vi "ReadQualisysFileInfo.vi"(4 "sortie d'erreur":errorcluster caption="entrée d'erreur", 7 "FichierQualisys":path) -> (0 "error out":errorcluster, 2 "horodatage":timestamp)   [LabVIEW 2015]
uses:
  <vilib>/Utility/miscctls.llb/LVDateTimeRec.ctl
panel:
  out "texte":string
  out "dt":dbl
  out "Freq":u32
  out "Noms des colonnes":string[](array[string])
  out "Noms des bodies":string[](array[string])
  out "NbBodies":u32
  out "NbCameras":u32
  out "NbFrames":u32
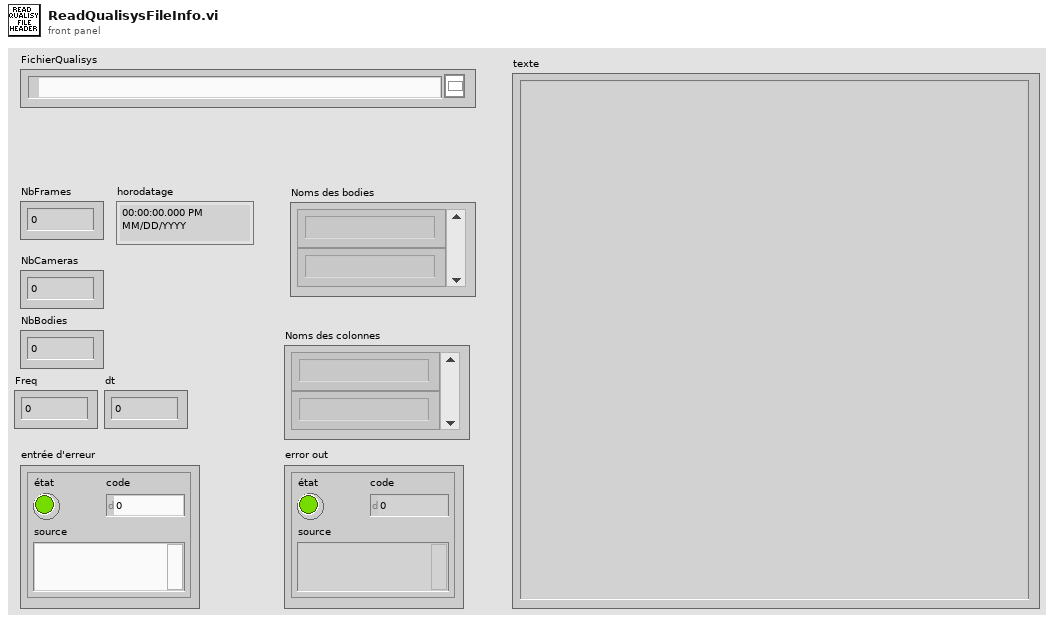
[diagram p1: front panel]
types:
  T1 = typedef "LVDateTimeRec.ctl" = cluster{"fractional second":dbl, "second":i32, "minute":i32, "hour":i32, "day of month":i32, "month":i32, "year":i32, "day of week":i32, "day of year":i32, "DST":i32}
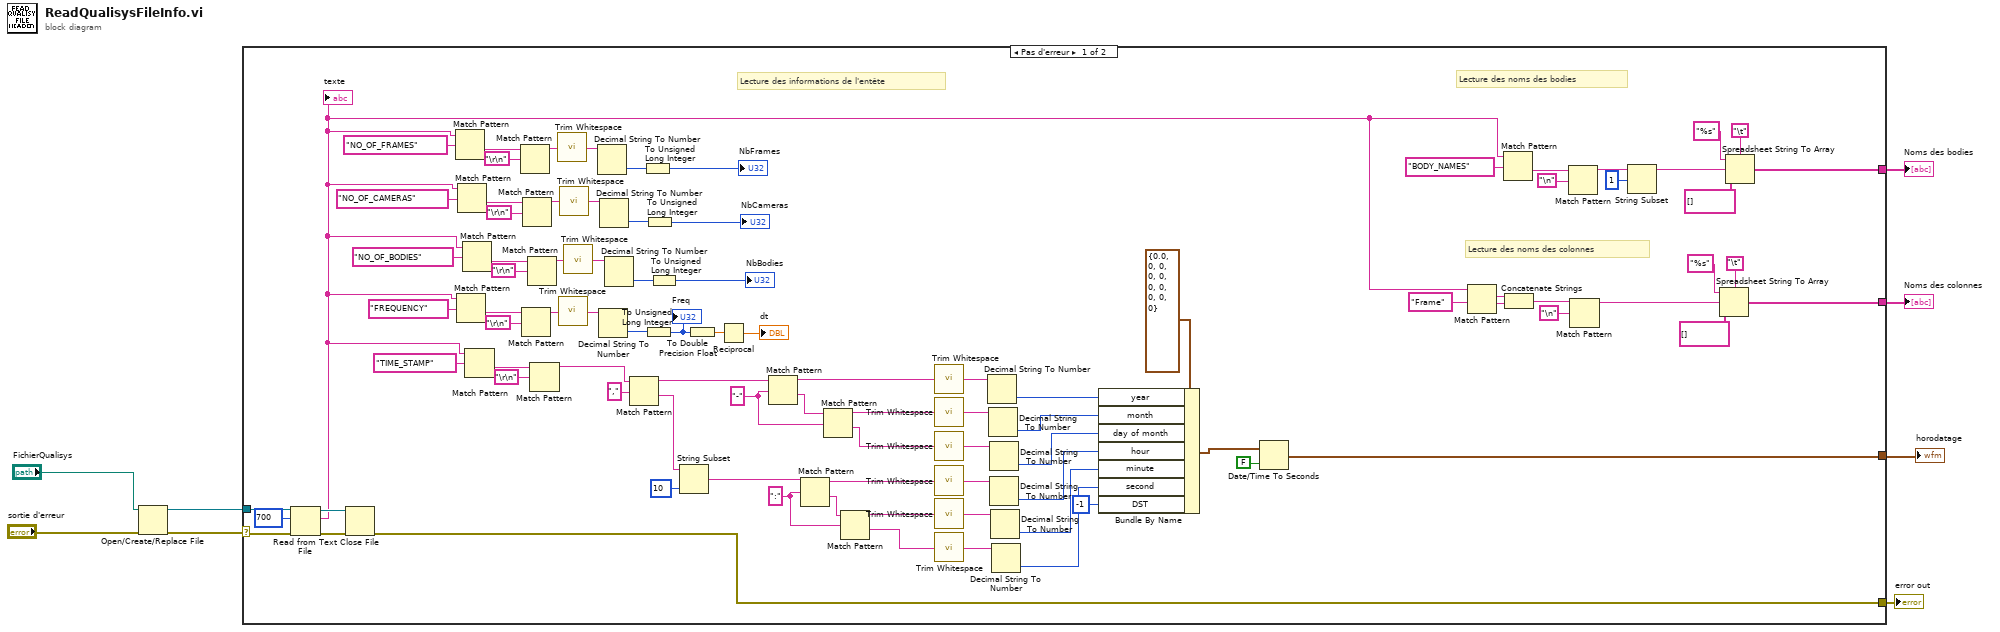
[diagram p0: block diagram]
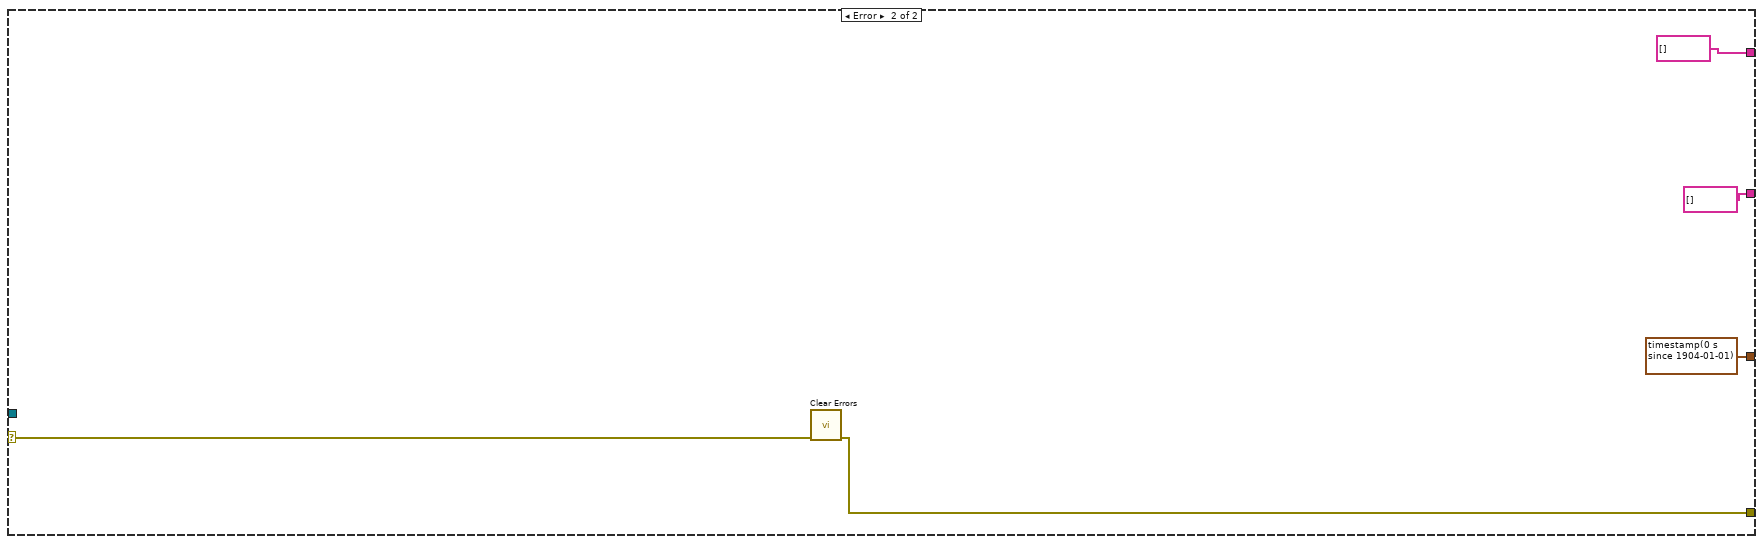
[diagram p2: hidden frame]
diagram:
  n1 = Open/Create/Replace File(file path (use dialog)="FichierQualisys", error in="sortie d'erreur") -> (refnum out=w5:refnum<file>, error out=w8:errorcluster)  [unwired: 4 in, 1 out]
  n2 = case shown="Pas d'erreur" w8 {
    selector: w8 -> [w99 w102]
    tunnel: w5 -> [w98 _]
    tunnel: [w15 w106] -> w1
    tunnel: [w12 timestamp(0 s since 1904-01-01) ("time stamp")] -> w2
    tunnel: [w14 string[] [] ("type de tableau (2D de dbl)")] -> w4
    tunnel: [w13 string[] [] ("type de tableau (2D de dbl)")] -> w3
    frame No Error {
      w57 = ":" ("expression régulière")
      w67 = "-" ("expression régulière")
      # "Lecture des noms des colonnes"
      # "Lecture des noms des bodies"
      # "Lecture des informations de l'entête"
      n3 = Read from Text File(file (use dialog)=w98, count=700 ("nombre"), error in=w99) -> (refnum out=w100:refnum<file>, text=w19:string, error out=w101:errorcluster)  [unwired: 1 in, 1 out]
      "texte" <- w19
      n4 = Close File(refnum=w100, error in=w101) -> (error out=w15:errorcluster)  [unwired: 1 out]
      n5 = Match Pattern(string=w19, regular expression="NO_OF_FRAMES" ("expression régulière")) -> (after substring=w95:string)  [unwired: 1 in, 3 out]
      n6 = Match Pattern(string=w19, regular expression="FREQUENCY" ("expression régulière")) -> (after substring=w22:string)  [unwired: 1 in, 3 out]
      n7 = Match Pattern(string=w19, regular expression="NO_OF_CAMERAS" ("expression régulière")) -> (after substring=w87:string)  [unwired: 1 in, 3 out]
      n8 = Match Pattern(string=w19, regular expression="NO_OF_BODIES" ("expression régulière")) -> (after substring=w82:string)  [unwired: 1 in, 3 out]
      n9 = Match Pattern(string=w19, regular expression="TIME_STAMP" ("expression régulière")) -> (after substring=w78:string)  [unwired: 1 in, 3 out]
      n10 = Match Pattern(string=w95, regular expression="\r\n") -> (before substring=w92:string)  [unwired: 1 in, 3 out]
      n11 = Match Pattern(string=w22, regular expression="\r\n") -> (before substring=w24:string)  [unwired: 1 in, 3 out]
      n12 = Match Pattern(string=w87, regular expression="\r\n") -> (before substring=w89:string)  [unwired: 1 in, 3 out]
      n13 = Match Pattern(string=w82, regular expression="\r\n") -> (before substring=w80:string)  [unwired: 1 in, 3 out]
      n14 = Match Pattern(string=w78, regular expression="\r\n") -> (before substring=w74:string)  [unwired: 1 in, 3 out]
      n15 = call <vilib>:"Trim Whitespace.vi"("string"=w92) -> ("trimmed string"=w91:string)  [unwired: 1 in]
      n16 = call <vilib>:"Trim Whitespace.vi"("string"=w24) -> ("trimmed string"=w25:string)  [unwired: 1 in]
      n17 = call <vilib>:"Trim Whitespace.vi"("string"=w89) -> ("trimmed string"=w90:string)  [unwired: 1 in]
      n18 = call <vilib>:"Trim Whitespace.vi"("string"=w80) -> ("trimmed string"=w79:string)  [unwired: 1 in]
      n19 = Decimal String To Number(string=w91) -> (number=w94:i32)  [unwired: 2 in, 1 out]
      n20 = Decimal String To Number(string=w25) -> (number=w23:i32)  [unwired: 2 in, 1 out]
      n21 = Decimal String To Number(string=w90) -> (number=w88:i32)  [unwired: 2 in, 1 out]
      n22 = Decimal String To Number(string=w79) -> (number=w81:i32)  [unwired: 2 in, 1 out]
      n23 = Match Pattern(string=w74, regular expression="," ("expression régulière")) -> (before substring=w69:string, after substring=w55:string)  [unwired: 1 in, 2 out]
      n24 = To Unsigned Long Integer(number=w94) -> (unsigned 32bit integer=→"NbFrames":u32)
      n25 = To Unsigned Long Integer(number=w23) -> (unsigned 32bit integer=w18:u32)
      "Freq" <- w18
      n26 = To Unsigned Long Integer(number=w88) -> (unsigned 32bit integer=→"NbCameras":u32)
      n27 = To Unsigned Long Integer(number=w81) -> (unsigned 32bit integer=→"NbBodies":u32)
      n28 = String Subset(string=w55, length (rest)=10 ("longueur (reste)")) -> (substring=w54:string)  [unwired: 1 in]
      n29 = To Double Precision Float(number=w18) -> (double precision float=w17:dbl)
      n30 = Reciprocal(x=w17) -> (1/x=→"dt":dbl)
      n31 = Match Pattern(string=w69, regular expression=w67) -> (before substring=w66:string, after substring=w68:string)  [unwired: 1 in, 2 out]
      n32 = Match Pattern(string=w54, regular expression=w57) -> (before substring=w58:string, after substring=w56:string)  [unwired: 1 in, 2 out]
      n33 = Match Pattern(string=w68, regular expression=w67) -> (before substring=w64:string, after substring=w63:string)  [unwired: 1 in, 2 out]
      n34 = Match Pattern(string=w56, regular expression=w57) -> (before substring=w59:string, after substring=w60:string)  [unwired: 1 in, 2 out]
      n35 = call <vilib>:"Trim Whitespace.vi"("string"=w66) -> ("trimmed string"=w49:string)  [unwired: 1 in]
      n36 = call <vilib>:"Trim Whitespace.vi"("string"=w64) -> ("trimmed string"=w48:string)  [unwired: 1 in]
      n37 = call <vilib>:"Trim Whitespace.vi"("string"=w63) -> ("trimmed string"=w47:string)  [unwired: 1 in]
      n38 = call <vilib>:"Trim Whitespace.vi"("string"=w58) -> ("trimmed string"=w46:string)  [unwired: 1 in]
      n39 = call <vilib>:"Trim Whitespace.vi"("string"=w59) -> ("trimmed string"=w45:string)  [unwired: 1 in]
      n40 = call <vilib>:"Trim Whitespace.vi"("string"=w60) -> ("trimmed string"=w44:string)  [unwired: 1 in]
      n41 = Decimal String To Number(string=w49) -> (number=w65:i32)  [unwired: 2 in, 1 out]
      n42 = Decimal String To Number(string=w48) -> (number=w62:i32)  [unwired: 2 in, 1 out]
      n43 = Decimal String To Number(string=w47) -> (number=w61:i32)  [unwired: 2 in, 1 out]
      n44 = Decimal String To Number(string=w46) -> (number=w52:i32)  [unwired: 2 in, 1 out]
      n45 = Decimal String To Number(string=w45) -> (number=w51:i32)  [unwired: 2 in, 1 out]
      n46 = Decimal String To Number(string=w44) -> (number=w50:i32)  [unwired: 2 in, 1 out]
      n47 = Bundle By Name(cluster=T1 {"fractional second"=0.0, "second"=0, "minute"=0, "hour"=0, "day of month"=0, "month"=0, "year"=0, "day of week"=0, "day of year"=0, "DST"=0} ("cluster date/heure"), "year"=w65, "month"=w62, "day of month"=w61, "hour"=w52, "minute"=w51, "second"=w50, "DST"=-1 ("day of year")) -> (w72:T1)
      n48 = Date/Time To Seconds(1:FALSE ("UTC (F)"), 2:w72) -> (0:w12:timestamp)
      n49 = Match Pattern(string=w19, regular expression="Frame" ("expression régulière")) -> (match substring=w29:string, after substring=w28:string)  [unwired: 1 in, 2 out]
      n50 = Match Pattern(string=w19, regular expression="BODY_NAMES" ("expression régulière")) -> (after substring=w43:string)  [unwired: 1 in, 3 out]
      n51 = Concatenate Strings(w29, w28) -> (w27:string)
      n52 = Match Pattern(string=w43, regular expression="\n") -> (before substring=w40:string)  [unwired: 1 in, 3 out]
      n53 = Match Pattern(string=w27, regular expression="\n") -> (before substring=w26:string)  [unwired: 1 in, 3 out]
      n54 = String Subset(string=w40, offset (0)=1) -> (substring=w36:string)  [unwired: 1 in]
      n55 = Spreadsheet String To Array(delimiter (Tab)="\t", format string="%s" ("chaîne de format"), spreadsheet string=w26, array type (2D Dbl)=string[] [] ("type de tableau (2D de dbl)")) -> (array=w14:string[])
      n56 = Spreadsheet String To Array(delimiter (Tab)="\t", format string="%s" ("chaîne de format"), spreadsheet string=w36, array type (2D Dbl)=string[] [] ("type de tableau (2D de dbl)")) -> (array=w13:string[])
    }
    frame Error {
      n57 = call <vilib>:"Clear Errors.vi"("error in (no error)"=w102) -> ("error out"=w106:errorcluster)  [unwired: 5 in, 1 out]
    }
  }
  "horodatage" <- w2
  "Noms des colonnes" <- w4
  "Noms des bodies" <- w3
  "error out" <- w1
